vi "LiftMain.vi"(8 "Boolean 2":bool, 9 "Boolean":bool, 10 "Input":dbl min=-1.0 max=1.0) -> ()   [LabVIEW 2016]
panel:
  out "Output":dbl
  in  "Invert?":bool
  in  "Enum":enum16{"Open", "Control"}(ring)
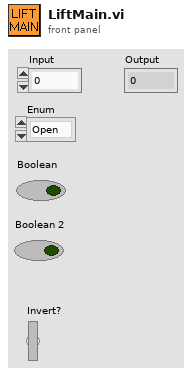
[diagram p1: front panel]
types:
  T1 = typedef "WPI_MotorControlDeviceRef.ctl" = cluster{"DeviceStatus":errorcluster, "Type":T2, "PWM":cluster{"PWM Channel":T3, "DeadBand":T4}, "CAN":cluster{"Device Number":u8, "SetOutput VI Ref":variant, "GetOutput VI Ref":variant, "Enable VI Ref":variant, "Disable VI Ref":variant, "Data":variant}, "Invert":bool}
  T2 = typedef "WPI_MotorControlType.ctl" = enum16{"PWM", "CAN"}
  T3 = typedef "FPGA_DIOPWMChannel.ctl" = enum8{"PWM 0", "PWM 1", "PWM 2", "PWM 3", "PWM 4", "PWM 5", "PWM 6", "PWM 7", "PWM 8", "PWM 9", "PWM MXP 0", "PWM MXP 1", "PWM MXP 2", "PWM MXP 3", "PWM MXP 4", "PWM MXP 5", "PWM MXP 6", "PWM MXP 7", "PWM MXP 8", "PWM MXP 9", "Invalid"}
  T4 = typedef "WPI_PWMDeadband.ctl" = cluster{"Name":string, "maxPositivePwm":i32, "minPositivePwm":i32, "centerPwm":i32, "maxNegativePwm":i32, "minNegativePwm":i32, "angularRange":u16}
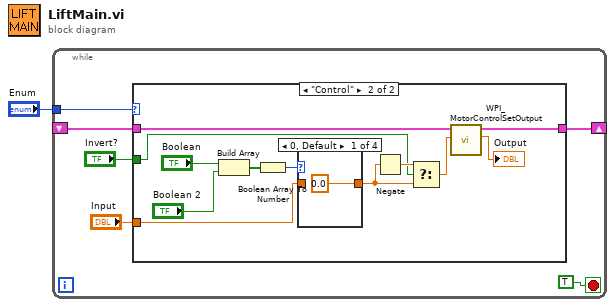
[diagram p0: block diagram]
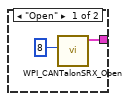
[diagram p2: hidden frame]
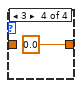
[diagram p5: hidden frame]
diagram:
  n1 = while {
    shift-right: [w5] -> _
    shift-left: _ -> [w4]
    tunnel: "Enum" -> [w6]
    stop <- TRUE stop-if-true
    n2 = case shown="\"Control\"" w6 {
      tunnel: [w9 w15] -> w5
      tunnel: w4 -> [_ w21]
      tunnel: "Input" -> [_ w16]
      tunnel: "Invert?" -> [_ w11]
      frame "Open" {
        n3 = call <vilib>:"WPI_CANTalonSRX_Open.vi"("Device Number"=u8 8) -> ("CAN Talon SRX Ref"=w9:T1)  [unwired: 9 in, 1 out]
      }
      frame "Control" {
        n4 = Build Array("Boolean", "Boolean 2") -> (w18:bool[])
        n5 = Boolean Array To Number(Boolean array=w18) -> (number=w17:u32)
        n6 = case shown="0, Default" w17 {
          tunnel: [0.0 w23 w24 0.0 ("Output")] -> w13
          tunnel: w16 -> [_ w23 w24 _]
          frame 0, Default {
          }
          frame 1 {
          }
          frame 2 {
          }
          frame 3 {
          }
        }
        n7 = Negate(x=w13) -> (-x=w14:dbl)
        n8 = Select(t=w14, s=w11, f=w13) -> (s? t:f=w12:dbl)
        n9 = call <vilib>:"WPI_MotorControlSetOutput.vi"("Output"=w12, "MotorControlDevRef"=w21) -> ("Motor Output"=→"Output":dbl, "MotorControlDevRef"=w15:T1)  [unwired: 7 in, 1 out]
      }
    }
  }
